vi "Create-client-channel.vi"(8 "error in (no error)":errorcluster, 10 "Client type":T1, 11 "ModComm in":T2) -> (0 "error out":errorcluster, 1 "Client ID":i32, 2 "Client channel":refnum<queue>, 3 "ModComm out":T2)   [LabVIEW 2013, in "Server.lvlib" / "Server.lvclass"]
uses:
  Server.lvclass
  Object-reference.ctl
  Messages/Sources/Message.lvclass
  Supported-module-types.ctl
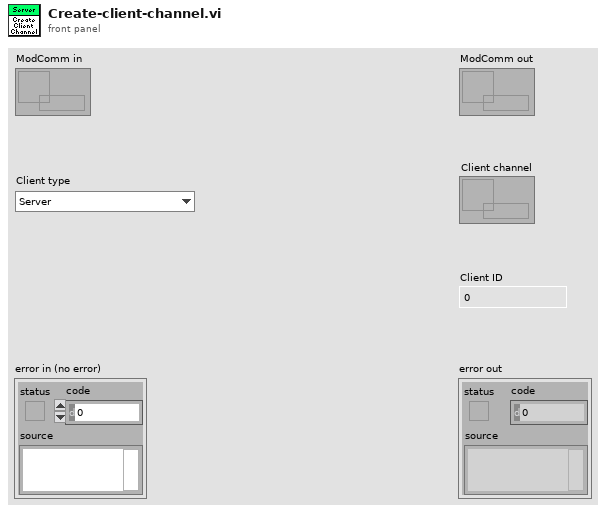
[diagram p1: front panel]
types:
  T1 = typedef "Server.lvlib/Server.lvclass/Supported-module-types.ctl" = enum16{"Server", "All", "BeamControl", "PowderDeposition", "StrategyParser", "CameraVision", "MaterialCharacterization", "StatusMonitor", "SLMSimulation", "LaserCharacterization"}
  T2 = typedef "Server.lvlib/Server.lvclass/Object-reference.ctl" = refnum<data-value>
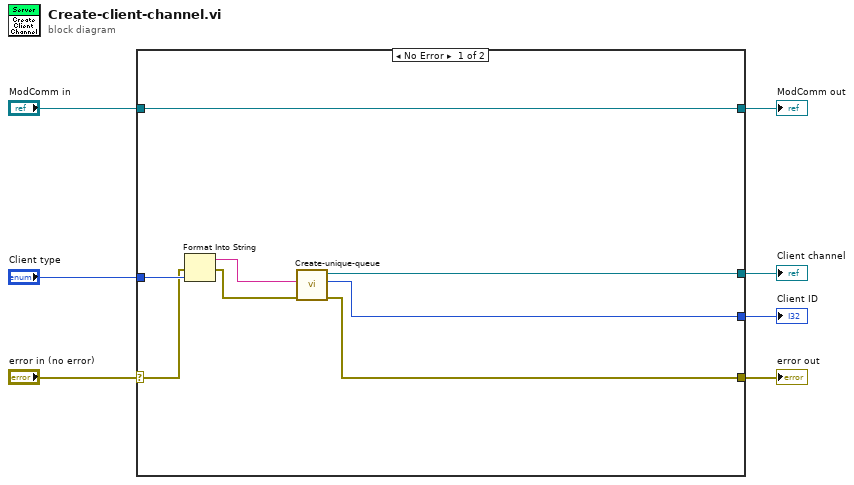
[diagram p0: block diagram]
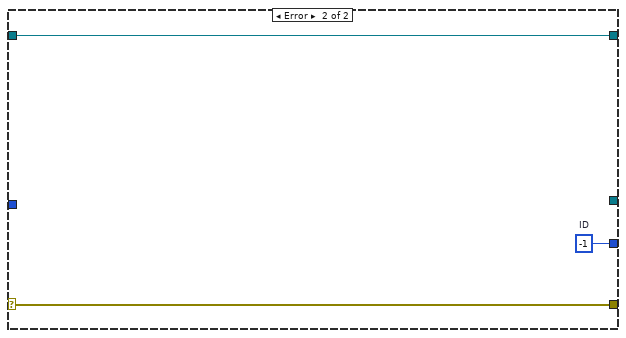
[diagram p2: hidden frame]
diagram:
  n1 = case shown="No Error" "error in (no error)" {
    selector: "error in (no error)" -> [w10 w18]
    tunnel: [w15 w18] -> w6
    tunnel: [w9 w17] -> w4
    tunnel: "ModComm in" -> [w9 w17]
    tunnel: [w14 _] -> w3
    tunnel: "Client type" -> [w13 _]
    tunnel: [w8 w16] -> w1
    frame No Error {
      n2 = Format Into String(error in=w10, w13) -> (resulting string=w12:string, error out=w11:errorcluster)  [unwired: 2 in]
      n3 = call "Create-unique-queue.vi"("error in (no error)"=w11, "Prefix"=w12) -> ("error out"=w15:errorcluster, "ID"=w8:i32, "Queue out"=w14:refnum<queue>)  [unwired: 7 in]
    }
    frame Error {
      w16 = -1  # ID
    }
  }
  "error out" <- w6
  "ModComm out" <- w4
  "Client channel" <- w3
  "Client ID" <- w1
